vi "T7MOD_Read_UINT16_Register.vi"(6 "Timeout":i32=10000, 8 "error in":errorcluster, 9 "LabJack UINT16 Register":i32=55110, 10 "Remote Port":u16=502, 11 "Remote IP Address":string="192.168.1.15") -> (0 "error out":errorcluster, 1 "Read At":timestamp, 2 "Raw Data Read":u16[](array[numeric]), 3 "Read UINT16":u16)   [LabVIEW 2018]
panel:
  # "Output"
  # "TCP Parameters"
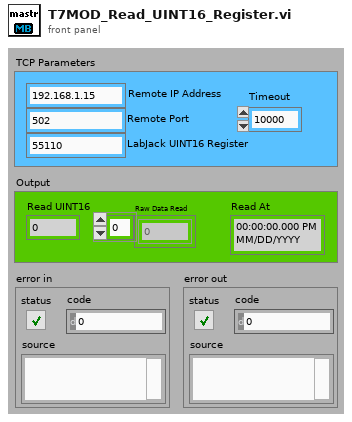
[diagram p1: front panel]
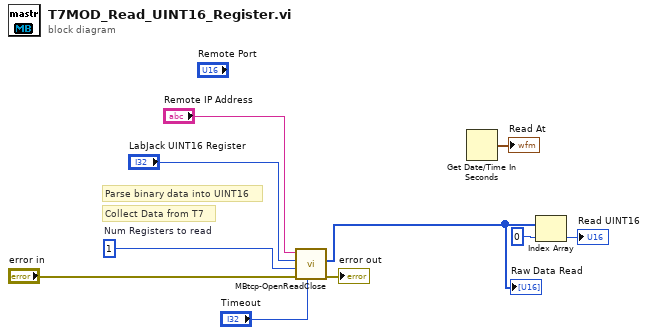
[diagram p0: block diagram]
diagram:
  w5 = 1  # Num Registers to read
  # "Parse binary data into UINT16"
  # "Collect Data from T7"
  n1 = call "MBtcp-OpenReadClose.vi"("Timeout (900)"="Timeout", "error in (no error)"="error in", "nRegisters"=w5, "RegisterAddr"="LabJack UINT16 Register", "IP Address(:port)"="Remote IP Address") -> ("error out"=→"error out":errorcluster, "16bitValues"=w1:u16[])  [unwired: 4 in, 1 out]
  "Raw Data Read" <- w1
  n2 = Get Date/Time In Seconds() -> (seconds since 1Jan1904=→"Read At":timestamp)
  n3 = Index Array(array=w1, index=0) -> (element=→"Read UINT16":u16)
